vi "cluster.vi"() -> ()   [LabVIEW 2019]
panel:
  out "source":string
  out "code":i32
  out "status":bool
  out "error out":errorcluster
  in  "error in (no error)":errorcluster
  out "output cluster 3":T1
  out "output cluster 2":T1
  out "output cluster":cluster{bool, dbl, string}
  out "Boolean 2":bool
  out "Boolean":bool
  in  "Cluster":T1
  # "CLUSTER ERROR"
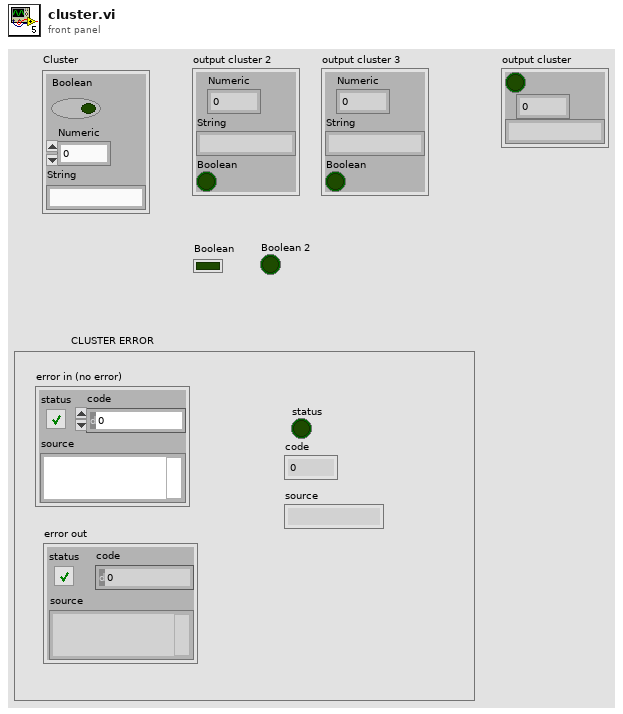
[diagram p1: front panel]
types:
  T1 = cluster{"Numeric":dbl, "String":string, "Boolean":bool}
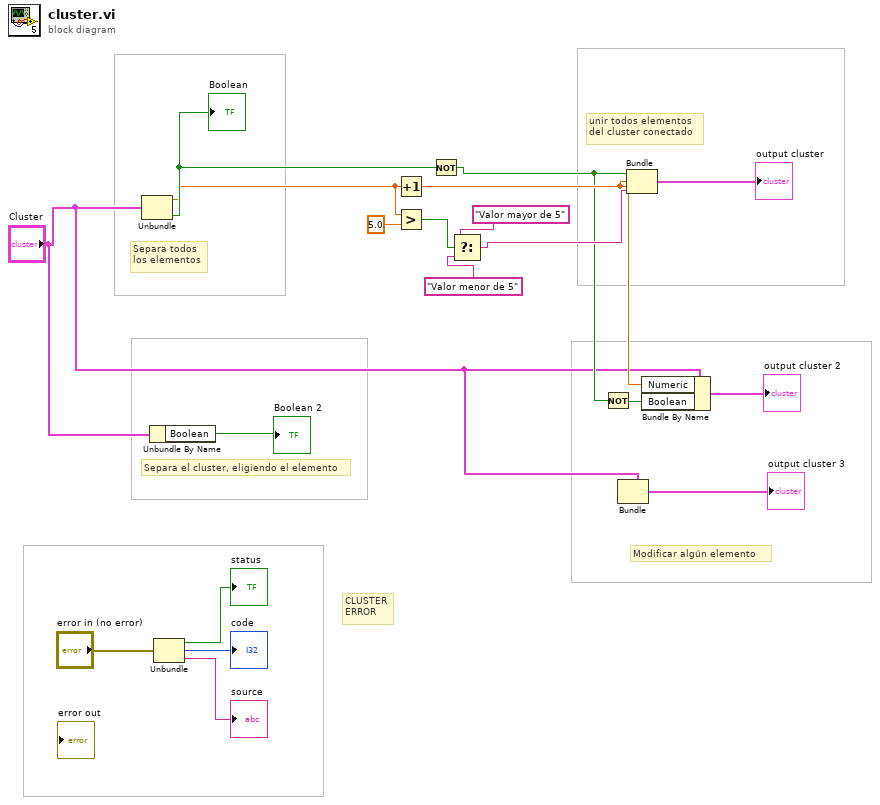
[diagram p0: block diagram]
diagram:
  # "Modificar algún elemento"
  # "CLUSTER\nERROR"
  # "unir todos elementos\ndel cluster conectado"
  # "Separa todos \nlos elementos"
  # "Separa el cluster, eligiendo el elemento"
  n1 = Unbundle "Unbundle"("Cluster") -> ("Numeric"=w17:dbl, "Boolean"=w18:bool)  [unwired: 1 out]
  "Boolean" <- w18
  n2 = Unbundle By Name "Unbundle By Name"("Cluster") -> ("Boolean"=→"Boolean 2":bool)
  n3 = Unbundle("error in (no error)") -> ("status"=→"status":bool, "code"=→"code":i32, "source"=→"source":string)
  n4 = Increment(x=w17) -> (x+1=w10:dbl)
  n5 = Greater?(x=w17, y=5.0) -> (0:w15:bool)
  n6 = Not(x=w18) -> (.not. x?=w8:bool)
  n7 = Select(t="Valor mayor de 5", s=w15, f="Valor menor de 5") -> (s? t:f=w12:string)
  n8 = Not(x=w8) -> (.not. x?=w9:bool)
  n9 = Bundle(cluster="Cluster") -> (→"output cluster 3":T1)  [unwired: 3 in]
  n10 = Bundle(w8, w10, w12) -> (→"output cluster":cluster{bool, dbl, string})  [unwired: 1 in]
  n11 = Bundle By Name(cluster="Cluster", "Numeric"=w10, "Boolean"=w9) -> (→"output cluster 2":T1)
